vi "SaveDataType.vi"(6 "Value 3":string[](array[string]), 7 "Value 2":string[](array[string]), 8 "Save Type":string(combo)=".csv", 9 "Value":i32, 10 "path":path, 11 "MulticolumnListbox输入":refnum<vi>) -> (3 "new file path (Not A Path if cancelled)":path)   [LabVIEW 2018]
uses:
  Global.vi
panel:
  out "添加的路径":path
  out "输出数组 2":string[](array[string])
  out "输出数组":string[](array[string])
  out "UUT OUT Data":string[][](array[string])
  # "D:\\Database\\CSV\\FAIL\\SN1(NA)20217993615.csv"
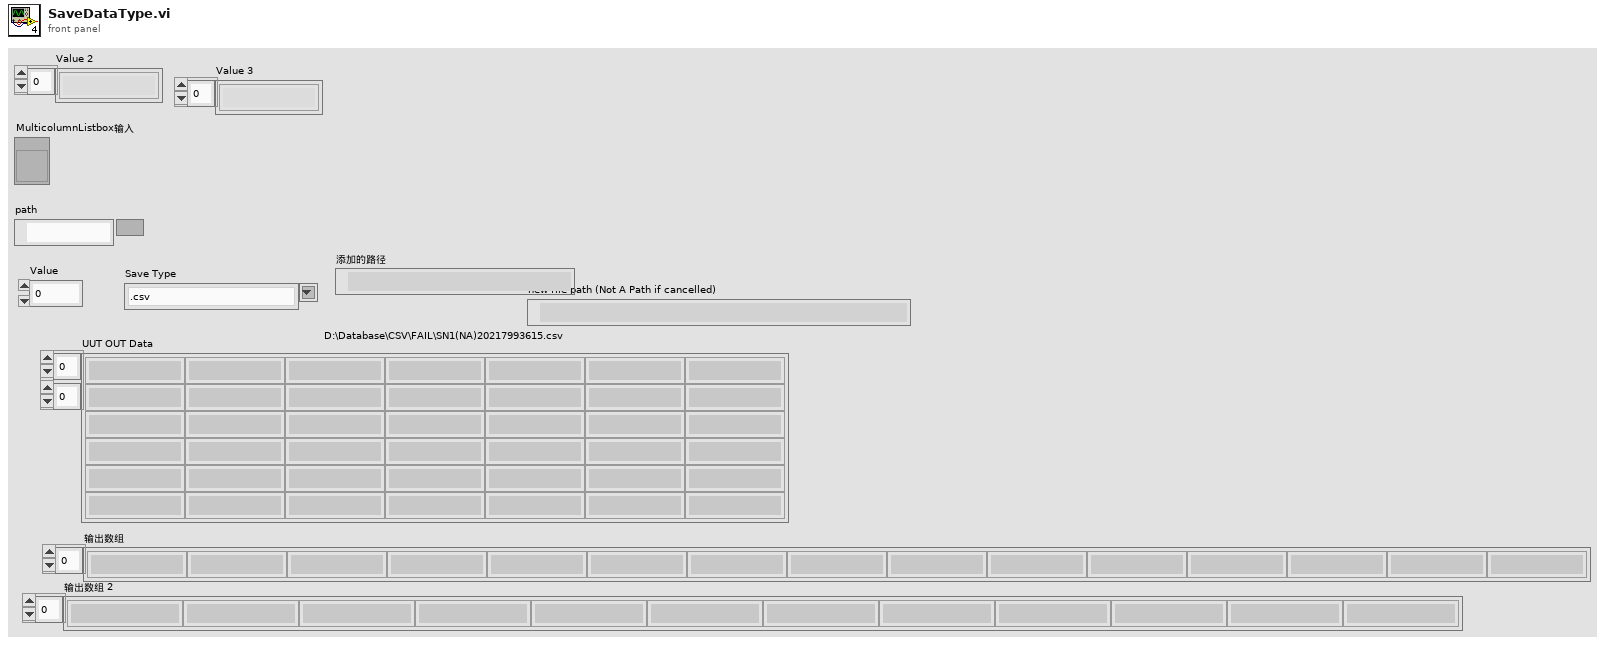
[diagram p1: front panel]
types:
  T1 = cluster{"Unit Timestamp":string, "SerialNumber":string, "StatusCode":string, "DateTimeStart":string, "DateTimeEnd":string, "TestProgramVersion":string, "TestFixtureNumber":string}
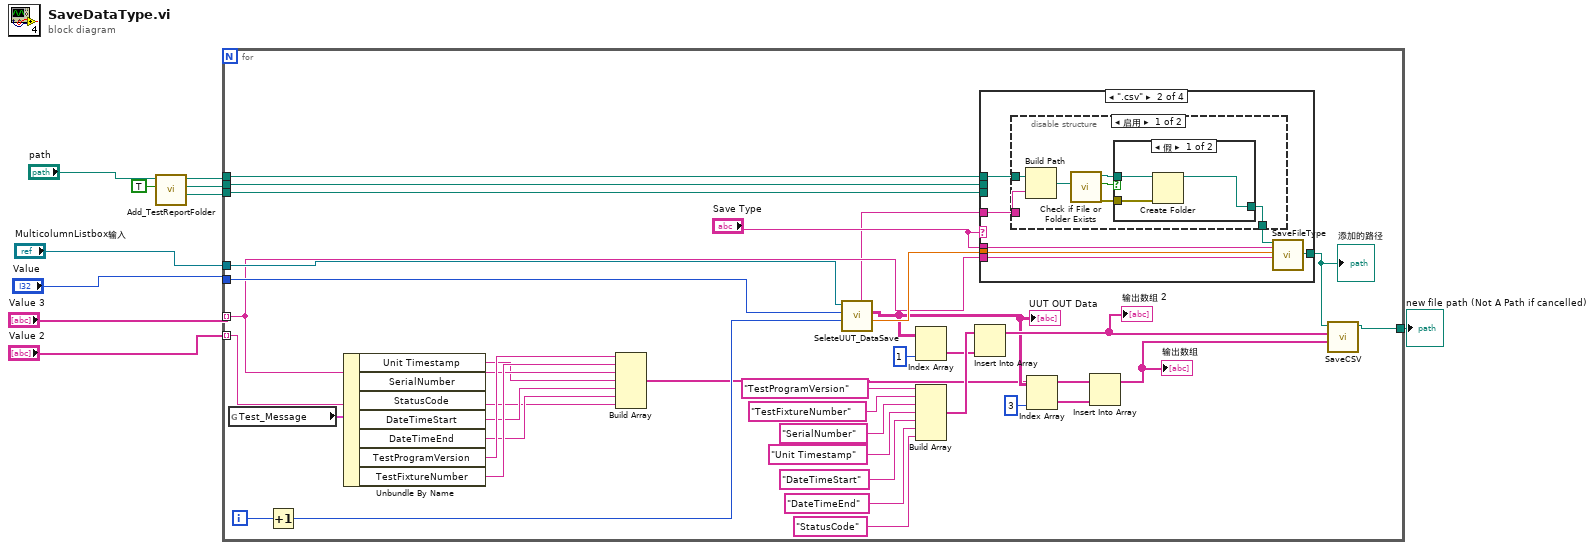
[diagram p0: block diagram]
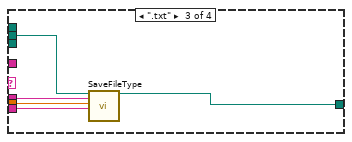
[diagram p5: hidden frame]
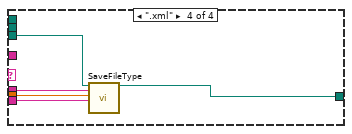
[diagram p6: hidden frame]
diagram:
  n1 = call "Add_TestReportFolder.vi"("是否新建多类文件夹"=TRUE, "path"="path") -> ("XLM path"=w9:path, "TXT path"=w8:path, "CSV path"=w7:path)  [unwired: 5 in, 2 out]
  n2 = for {
    tunnel: "Value 3" -> [w23] mode=indexing
    tunnel: "Value 2" -> [w19] mode=indexing
    tunnel: "MulticolumnListbox输入" -> [w43]
    tunnel: w7 -> [w42]
    tunnel: w8 -> [w15]
    tunnel: w9 -> [w14]
    tunnel: "Value" -> [w27]
    tunnel: [w16] -> w2
    i -> [w46]
    n3 = global read "Global.vi" "Test_Message"() -> (w26:T1)
    n4 = Increment(x=w46) -> (x+1=w45:i32)
    n5 = Unbundle By Name(w26) -> ("Unit Timestamp"=w22:string, "DateTimeStart"=w21:string, "DateTimeEnd"=w20:string, "TestProgramVersion"=w25:string, "TestFixtureNumber"=w24:string)  [unwired: 2 out]
    n6 = Build Array(w25, w24, w23, w22, w21, w20, w19) -> (w18:string[])
    n7 = call "SeleteUUT_DataSave.vi"("选择测试板数据"=w45, "测试步数"=w27, "real report 3"=w43) -> ("选择测试板数据 OUT"=w44:dbl, "UUT OUT Data"=w29:string[][], "PASS/FAIL"=w11:string)  [unwired: 5 in, 1 out]
    "UUT OUT Data" <- w29
    n8 = Index Array(array=w29, index (col)=1 ("禁用的索引 (列)")) -> (element=w32:string[])  [unwired: 1 in]
    n9 = Build Array("TestProgramVersion", "TestFixtureNumber", "SerialNumber", "Unit Timestamp", "DateTimeStart", "DateTimeEnd", "StatusCode") -> (w33:string[])
    n10 = Insert Into Array(array=w33, new element=w32) -> (w31:string[])  [unwired: 1 in]
    "输出数组 2" <- w31
    n11 = case shown="\".csv\"" "Save Type" {
      tunnel: "Save Type" -> [_ w53 w70 w75]
      tunnel: w44 -> [_ w52 w69 w74]
      tunnel: w42 -> [_ w49 _ _]
      tunnel: [_ w51 w68 w73] -> w41
      tunnel: w23 -> [_ w50 w67 w72]
      tunnel: w15 -> [_ _ w66 _]
      tunnel: w14 -> [_ _ _ w71]
      tunnel: w11 -> [_ w48 _ _]
      frame "假", Default {
      }
      frame ".csv" {
        n12 = disable-structure shown="启用" {
          disable-tunnel: w49 -> [w60 w65]
          disable-tunnel: w48 -> [w59 _]
          disable-tunnel: [w58 w65] -> w47
          frame Enabled {
            n13 = Build Path(base path=w60, name or relative path=w59) -> (appended path=w56:path)
            n14 = call <vilib>:"Check if File or Folder Exists.vi"("path"=w56) -> ("error out"=w57:errorcluster, "file or folder exists?"=w54:bool, "dup path"=w55:path)  [unwired: 8 in]
            n15 = case shown="假" w54 {
              tunnel: [w63 w64] -> w58
              tunnel: w57 -> [w62 _]
              tunnel: w55 -> [w61 w64]
              frame False {
                n16 = Create Folder(path (use dialog)=w61, error in=w62) -> (created path=w63:path)  [unwired: 1 in, 2 out]
              }
              frame True {
              }
            }
          }
          frame Disabled {
          }
        }
        n17 = call "SaveFileType.vi"("基路径"=w47, "Save Type"=w53, "数值"=w52, "SN INPUT"=w50) -> ("添加的路径"=w51:path)  [unwired: 13 in, 2 out]
      }
      frame ".txt" {
        n18 = call "SaveFileType.vi"("基路径"=w66, "Save Type"=w70, "数值"=w69, "SN INPUT"=w67) -> ("添加的路径"=w68:path)  [unwired: 13 in, 2 out]
      }
      frame ".xml" {
        n19 = call "SaveFileType.vi"("基路径"=w71, "Save Type"=w75, "数值"=w74, "SN INPUT"=w72) -> ("添加的路径"=w73:path)  [unwired: 13 in, 2 out]
      }
    }
    "添加的路径" <- w41
    n20 = Index Array(array=w29, index (col)=3 ("禁用的索引 (列)")) -> (element=w17:string[])  [unwired: 1 in]
    n21 = Insert Into Array(array=w18, new element=w17) -> (w28:string[])  [unwired: 1 in]
    "输出数组" <- w28
    n22 = call "SaveCSV.vi"("数据行"=w28, "表头"=w31, "Savepath"=w41) -> ("new file path (Not A Path if cancelled)"=w16:path)  [unwired: 8 in]
  }
  "new file path (Not A Path if cancelled)" <- w2
